vi "Untitled 2 (SubVI).vi"(8 "error in":errorcluster, 10 "limit":dbl, 11 "timerstate":T1) -> (0 "error out":errorcluster, 2 "limit reached":bool, 3 "elapsed":dbl)   [LabVIEW 2015]
uses:
  controls/timerstate.ctl
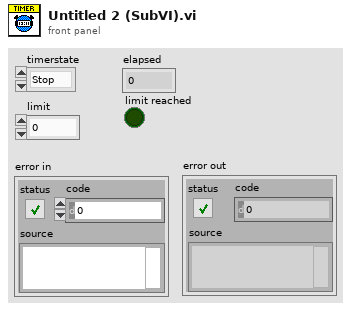
[diagram p1: front panel]
types:
  T1 = typedef "timerstate.ctl" = enum16{"Stop", "Pause", "Start"}
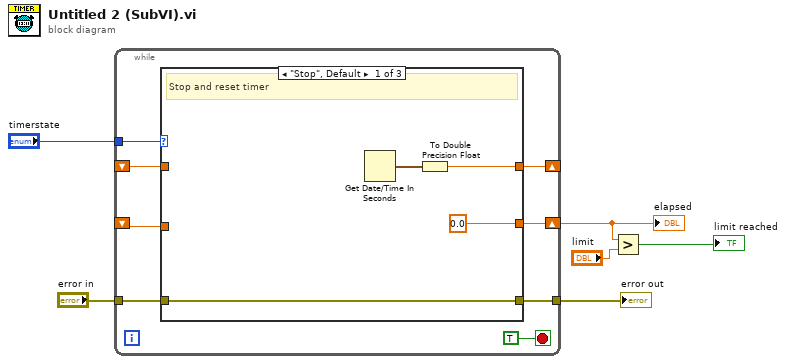
[diagram p0: block diagram]
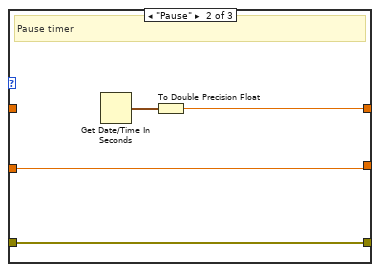
[diagram p2: hidden frame]
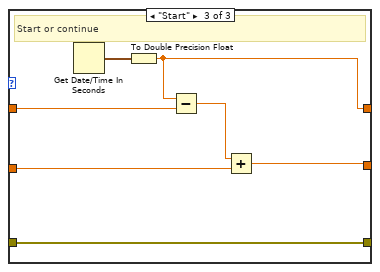
[diagram p3: hidden frame]
diagram:
  n1 = while {
    tunnel: "timerstate" -> [w13]
    shift-right: [w12] -> _
    shift-left: _ -> [w10]
    shift-right: [w11] -> w4
    shift-left: _ -> [w9]
    tunnel: "error in" -> [w8]
    tunnel: [w7] -> w1
    stop <- TRUE stop-if-true
    n2 = case shown="\"Stop\", Default" w13 {
      tunnel: [w17 w20 w28] -> w12
      tunnel: [0.0 w22 w24] -> w11
      tunnel: w10 -> [_ _ w27]
      tunnel: w9 -> [_ w22 w25]
      tunnel: w8 -> [w15 w19 w23]
      tunnel: [w15 w19 w23] -> w7
      frame "Stop", Default {
        # "Stop and reset timer"
        n3 = Get Date/Time In Seconds() -> (seconds since 1Jan1904=w18:timestamp)
        n4 = To Double Precision Float(number=w18) -> (double precision float=w17:dbl)
      }
      frame "Pause" {
        # "Pause timer"
        n5 = Get Date/Time In Seconds() -> (seconds since 1Jan1904=w21:timestamp)
        n6 = To Double Precision Float(number=w21) -> (double precision float=w20:dbl)
      }
      frame "Start" {
        # "Start or continue"
        n7 = Get Date/Time In Seconds() -> (seconds since 1Jan1904=w29:timestamp)
        n8 = To Double Precision Float(number=w29) -> (double precision float=w28:dbl)
        n9 = Subtract(x=w28, y=w27) -> (x-y=w26:dbl)
        n10 = Add(x=w26, y=w25) -> (x+y=w24:dbl)
      }
    }
  }
  "elapsed" <- w4
  "error out" <- w1
  n11 = Greater?(x=w4, y="limit") -> (0:→"limit reached":bool)
